vi "ID Manager.vi"(7 "action (Increment)":T1, 8 "error in":errorcluster, 11 "manual ID":i32) -> (0 "error out":errorcluster, 3 "ID out":i32)   [LabVIEW 2020, in "Ballard_1553_Hardware_ni.lvlib"]
uses:
  Ballard_1553_Hardware_ni.lvlib
  _typedefs/idManager_action.ctl
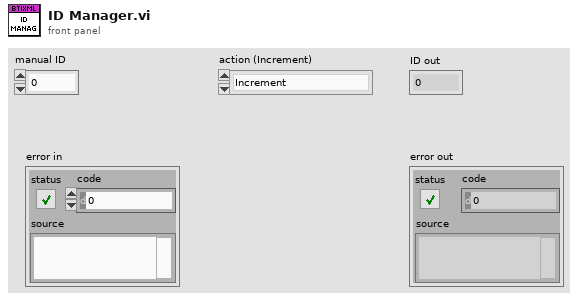
[diagram p1: front panel]
types:
  T1 = typedef "Ballard_1553_Hardware_ni.lvlib/idManager_action.ctl" = enum16{"Increment", "Get", "Set"}
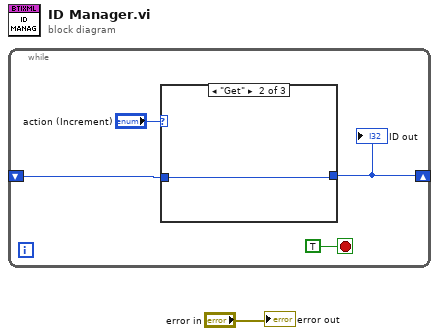
[diagram p0: block diagram]
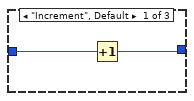
[diagram p2: hidden frame]
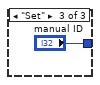
[diagram p3: hidden frame]
diagram:
  n1 = while {
    shift-right: [w3] -> _
    shift-left: _ -> [w2]
    stop <- TRUE stop-if-true
    n2 = case shown="\"Get\"" "action (Increment)" {
      tunnel: [w6 w8 "manual ID"] -> w3
      tunnel: w2 -> [w7 w8 _]
      frame "Increment", Default {
        n3 = Increment(x=w7) -> (x+1=w6:i32)
      }
      frame "Get" {
      }
      frame "Set" {
      }
    }
    "ID out" <- w3
  }
  "error out" <- "error in"
